vi "Write New Line.vi"(8 "error in (no error)":errorcluster, 9 "Indent ? ( F)":bool, 10 "New Line":string, 11 "Text":string) -> (0 "error out":errorcluster, 3 "Text (out)":string)   [LabVIEW 2017, in "WebServiceImporter.lvlib" / "Main Panel.lvlib" / "Preview.lvlib"]
uses:
  <vilib>/Platform/WebService/Main Panel/Pages/Preview/Preview.lvlib
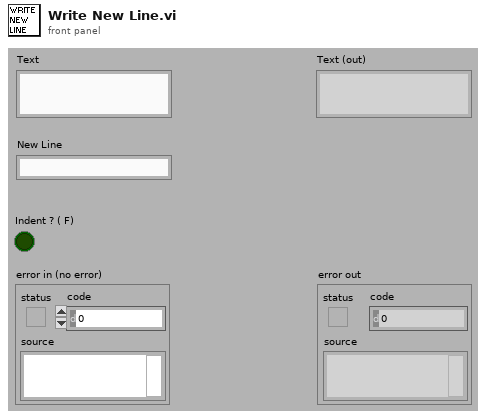
[diagram p1: front panel]
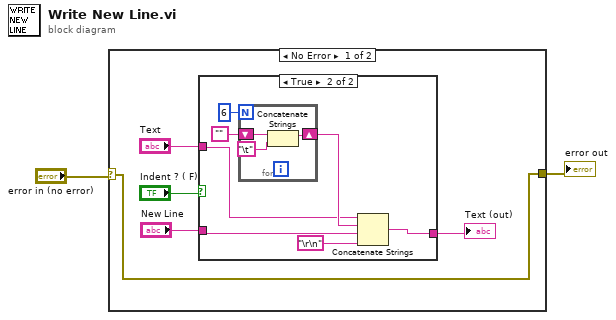
[diagram p0: block diagram]
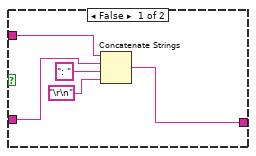
[diagram p2: hidden frame]
diagram:
  n1 = case shown="No Error" "error in (no error)" {
    selector: "error in (no error)" -> [w5 w23]
    tunnel: [w5 w23] -> w1
    frame No Error {
      n2 = case shown="True" "Indent ? ( F)" {
        tunnel: "Text" -> [w9 w14]
        tunnel: [w10 w15] -> w4
        tunnel: "New Line" -> [w8 w13]
        frame False {
          n3 = Concatenate Strings(w9, w8, ": ", "\r\n") -> (w10:string)
        }
        frame True {
          n4 = for {
            N: 6 -> [_]
            shift-right: [w20] -> w17
            shift-left: "" -> [w22]
            n5 = Concatenate Strings(w22, "\t") -> (w20:string)
          }
          n6 = Concatenate Strings(w14, w17, w13, "\r\n") -> (w15:string)
        }
      }
      "Text (out)" <- w4
    }
    frame Error {
    }
  }
  "error out" <- w1
